vi "Main.vi"() -> ()   [LabVIEW 2013]
doc: "Diese Vorlage dient zur Erzeugung eines Entwurfsmusters für einen einfachen Zustandsautomaten. Jeder Zustand führt einen bestimmten Blockdiagrammabschnitt aus und ermittelt dann den nächsten Zustand."
uses:
  controls/State.ctl
  controls/Data.ctl
  res/classes/Datastructure/Report/Report.lvclass
  res/classes/Devices/emTestCWS500N/EMTestCWS500N.lvclass
  res/classes/Devices/CEG4500/CEG4500.lvclass
  res/classes/Devices/Tektronix RSA5106A/Tektronix RSA5106A.lvclass
  res/classes/Devices/DeviceInterface/Devices.ctl
  res/classes/Tests/TestInterface/Tests.ctl
  res/vis/Tabs.ctl
  res/vis/ESD Pistol.lvclass
  <vilib>/event_ctls.llb/eventvkey.ctl
  res/classes/Datastructure/Norm/Norm.lvclass
  res/classes/Datastructure/Test/Test.lvclass
  <vilib>/Utility/error.llb/DialogType.ctl
  res/classes/Datastructure/Setup/Setup.lvclass
  res/vis/DeviceAddEdit.vi
  res/vis/Versuchsaufbau bearbeiten.vi
  res/vis/Test bearbeiten.vi
  res/lib/DataCreation.lvlib
  res/lib/Utilities.lvlib
  res/lib/EMV-Test.lvlib
  res/lib/TreeRepresentation.lvlib
  res/lib/XML.lvlib
  res/lib/TempHygro.lvlib
panel:
  out "running":bool=TRUE
  in  "error in (no error)":errorcluster
  out "COM-Port Refs":refnum<vi>[](array[refnum])
  out "Normen":string[](array[string])
  out "APPDATA":string
  out "return code":i32 caption="Fehlercode"
  out "standard error":string caption="Standardfehler"
  out "standard output":string caption="Standardausgabe"
  in  "Tab Control":T1(tab)
  in  "Button:Beenden":bool
  in  "Button:Start:HF-Felder":bool
  in  "Button:Start:Spannungseinbruch":bool
  in  "Button:Start:Surge":bool
  in  "Button:Start:ESD":bool
  in  "Button:Start:Burst":bool
  in  "Button:Start:Störaussendung":bool
  in  "Button:save Report":bool caption="Blank Button"
  in  "Button:load Report":bool caption="Blank Button"
  in  "Button:create Pdf":bool caption="Blank Button"
  in  "Debug":bool
  in  "Tree":string(tree)
  in  "Bild-Qualität ( 0 = schlechteste, 1 = beste)":dbl(slide)=0.4954128440366973 min=0.0 max=1.0 scale=0.0..1.0
  in  "Kalibrierung CDN":bool
  in  "Tektronix RSA5106A":refnum<visa-resource-name>="COM4"
  in  "CEG 4500":refnum<visa-resource-name>="COM13"
  in  "emTestCWS500N1":refnum<visa-resource-name>="COM5"
  in  "wait until completion? (T)":bool=TRUE
  in  "Path":path=path "C:/Windows/System32"
  # "COM-Ports"
  # "Pdf-Report"
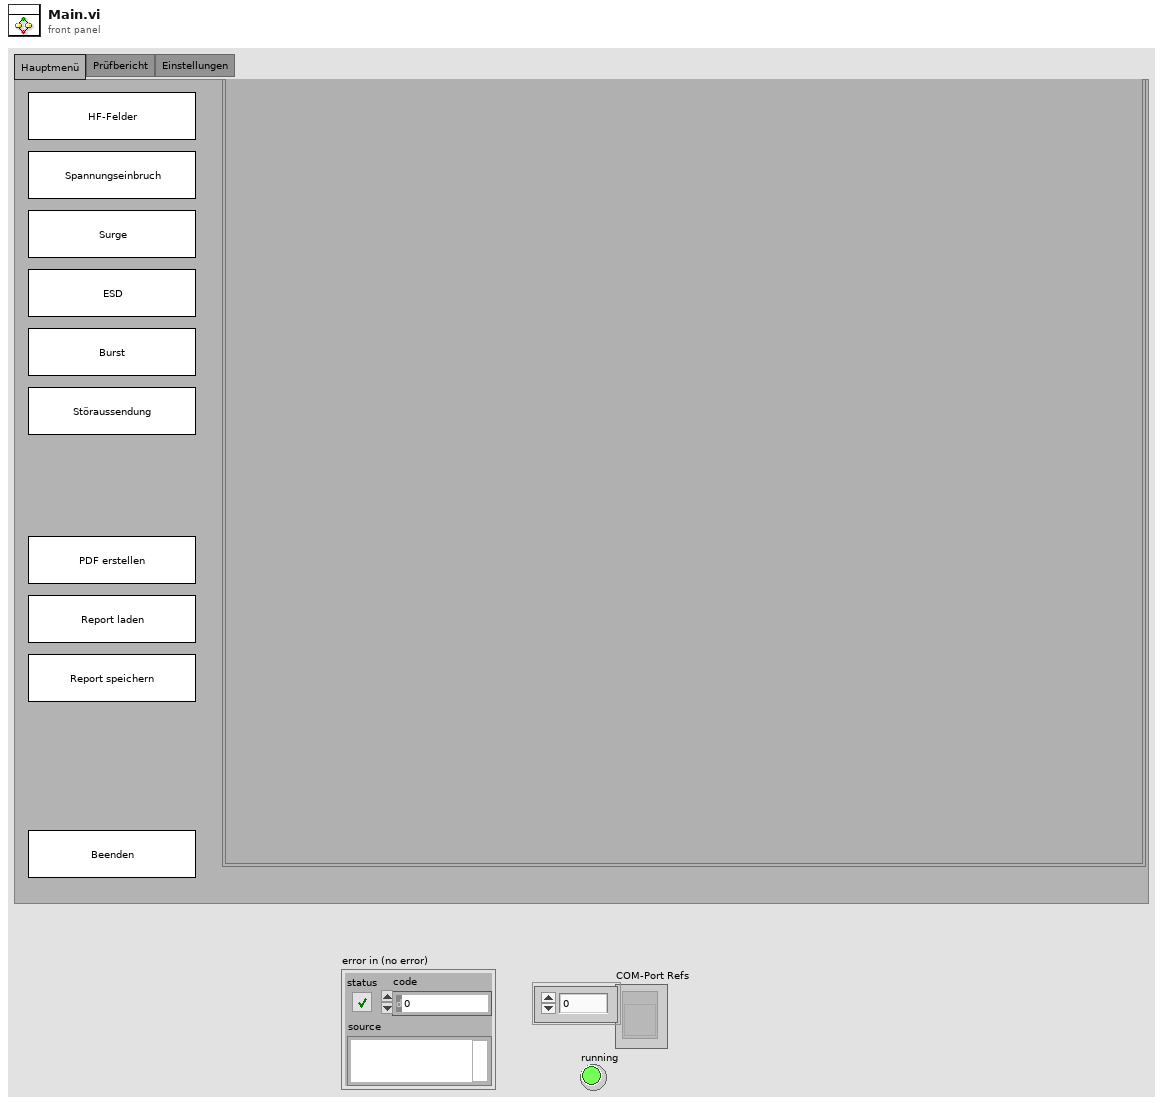
[diagram p1: front panel]
types:
  T1 = enum32{"Hauptmenü", "Prüfbericht", "Einstellungen"}
  T2 = typedef "Data.ctl" = cluster{"Report.lvclass":refnum<class "Report.lvclass">, "Norm":string, "last State":T3, "Norm ID":i32, "parameter":string[][], "EMTestCWS500N.lvclass":refnum<class "EMTestCWS500N.lvclass">, "CEG4500.lvclass":refnum<class "CEG4500.lvclass">, "Tektronix RSA5106A.lvclass":refnum<class "Tektronix RSA5106A.lvclass">, "erfolgreich":bool, "log":string, "Kommentar":string, "Device Enum":T4, "Test Enum":T5, "debug":bool, "tab":T6, "ESD Pistol.lvclass":refnum<class "ESD Pistol.lvclass">, "SubPnl Refnum":refnum<vi>, "TabCtl Refnum":refnum<vi>, "ButtonsEinblenden?":bool, "VKey":T7}
  T3 = typedef "State.ctl" = enum16{"create Pdf", "edit Report", "load Report", "save Report", "do Test", "CDN Kalibrierung", "enter Report Parameters", "new Test", "Protokoll", "read Tree", "update Tree", "Fehler", "Initialize", "Wait for Event", "Exit"}
  T4 = typedef "Devices.ctl" = enum16{"unbekannt", "ESD Pistol", "Tektronix RSA5106A", "emTestCWS500N", "CEG-4500"}
  T5 = typedef "Tests.ctl" = enum16{"unbekannt", "Störaussendung", "Burst", "ESD", "Surge", "Spannungseinbruch", "HF-Felder"}
  T6 = typedef "Tabs.ctl" = enum32{"Hauptmenü", "Prüfbericht", "Einstellungen"}
  T7 = typedef "eventvkey.ctl" = enum16{"ASCII", "Enter", "Return", "Shift", "Ctrl", "Alt", "Cmd", "Opt", "Caps", "NumLock", "Clear", "Break", "Up", "Down", "Left", "Right", "Insert", "Delete", "Home", "End", "PageUp", "PageDown", "Escape", "Help", "Pause", "ScrollLock", "F1", "F2", "F3", "F4", "F5", "F6", "F7", "F8", "F9", "F10", "F11", "F12", "F13", "F14", "F15", "F16", "F17", "F18", "F19", "F20", "F21", "F22", "F23", "F24", "Play", "VolumeUp", "VolumeDown", "Mute", "Two Byte Char"}
  T8 = enum8{"Enabled", "Disabled", "Disabled and Grayed Out"}
  T9 = typedef "DialogType.ctl" = u16
  T10 = enum16{"Left Button", "Center Button", "Right Button", "Window Close"}
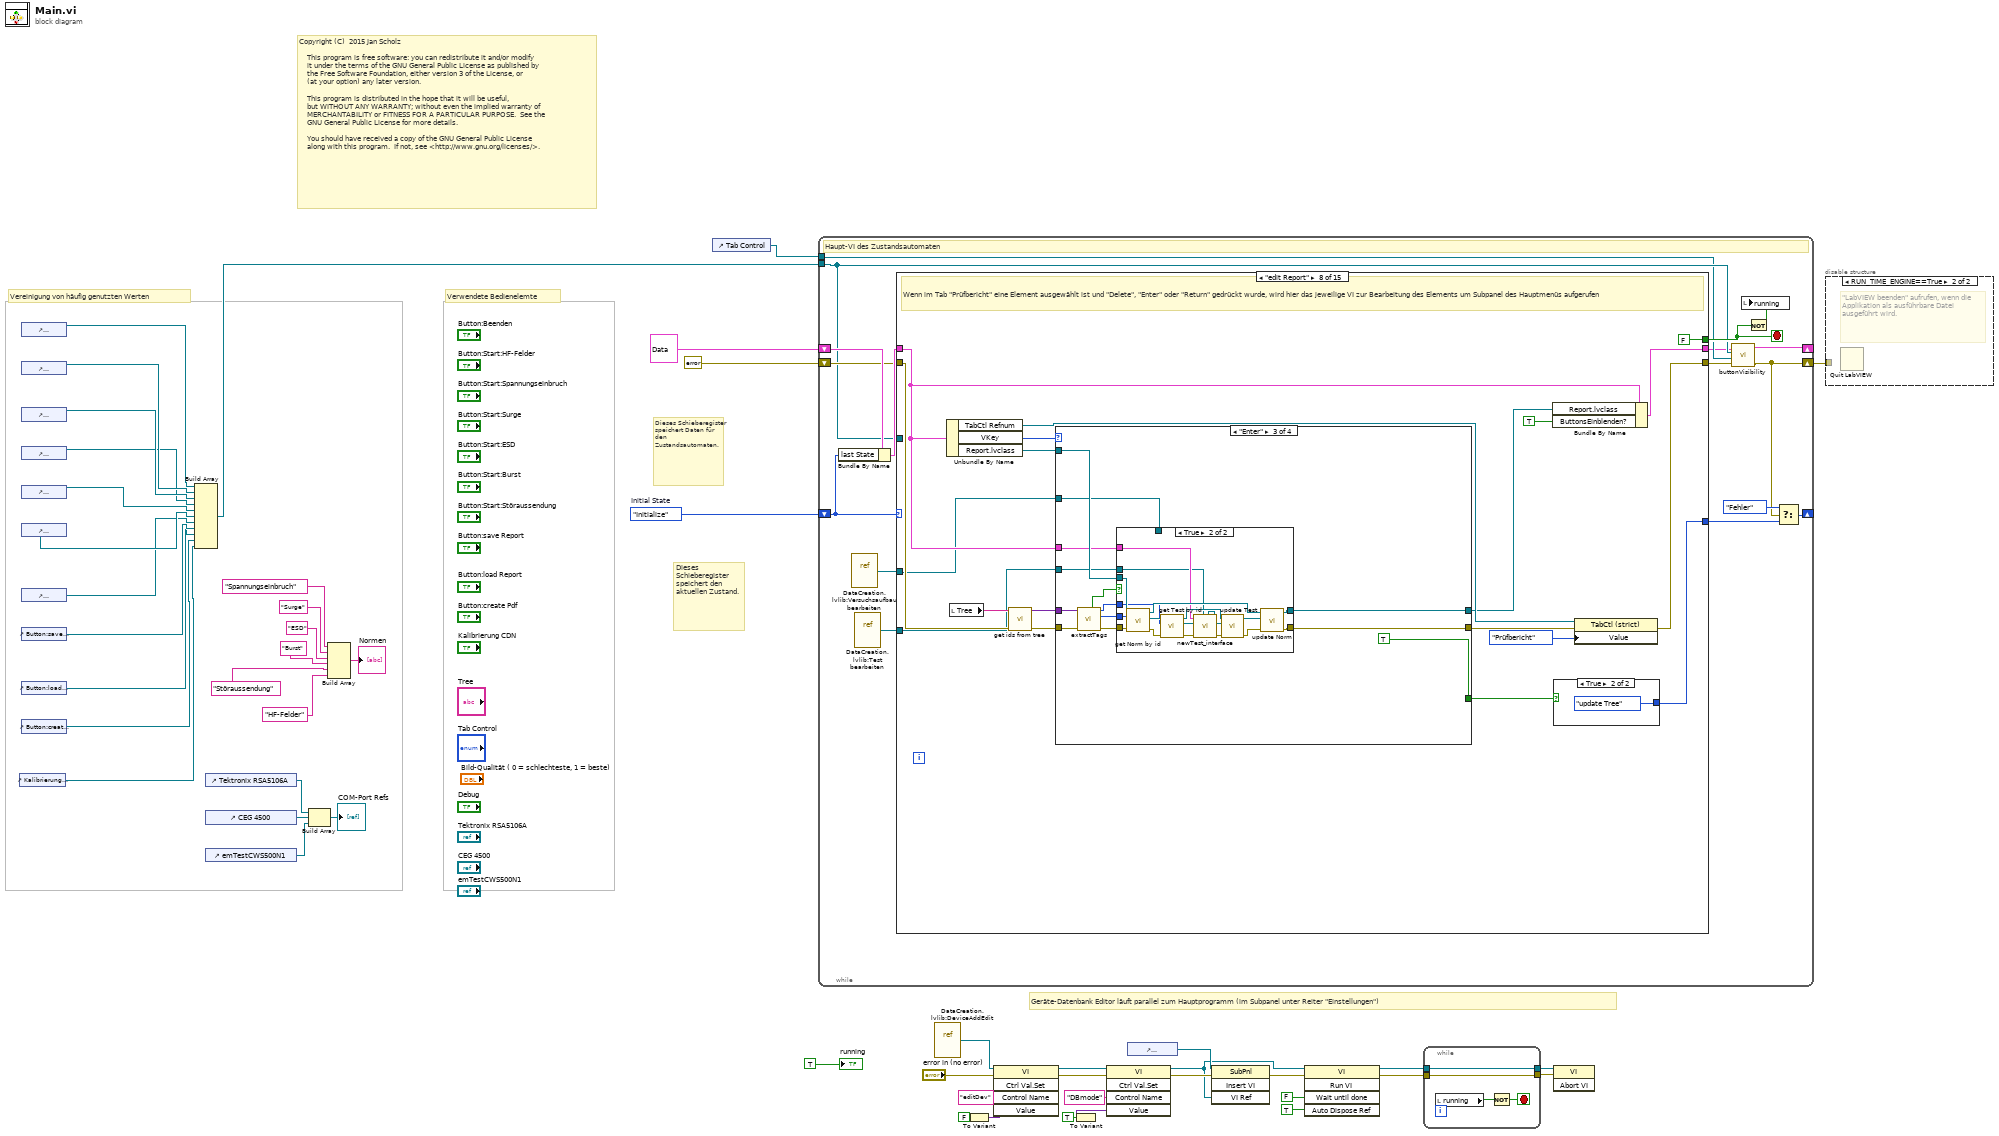
[diagram p0: block diagram]
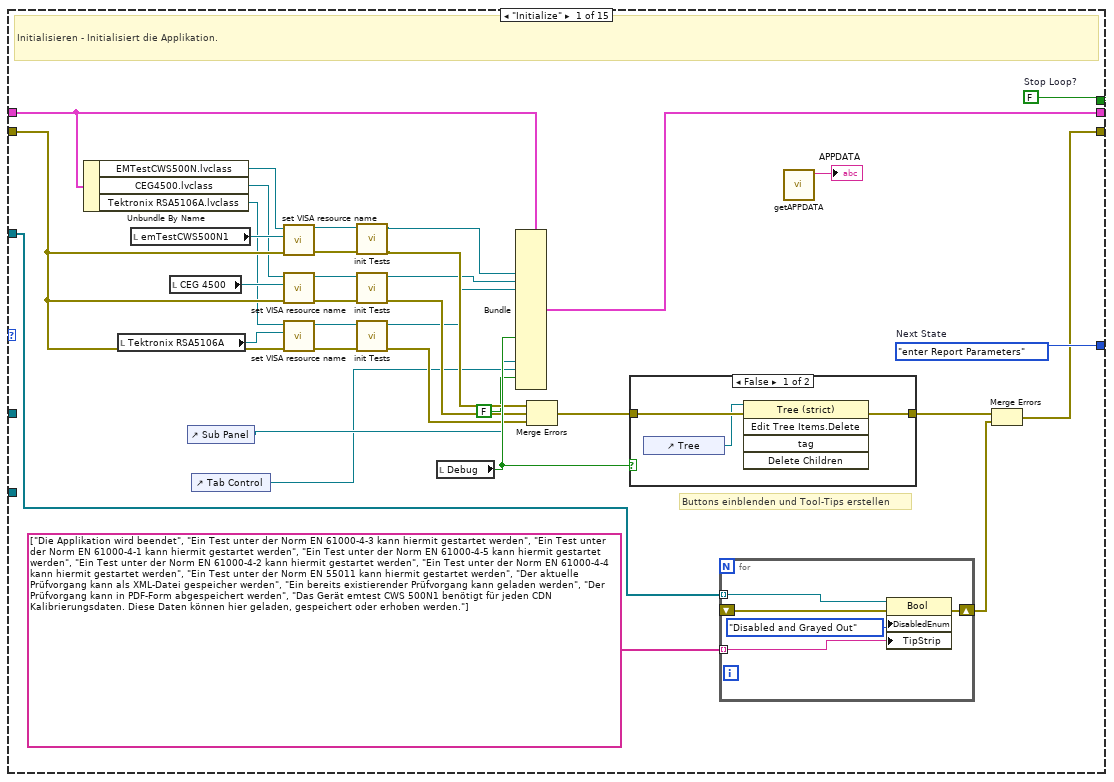
[diagram p3: hidden frame]
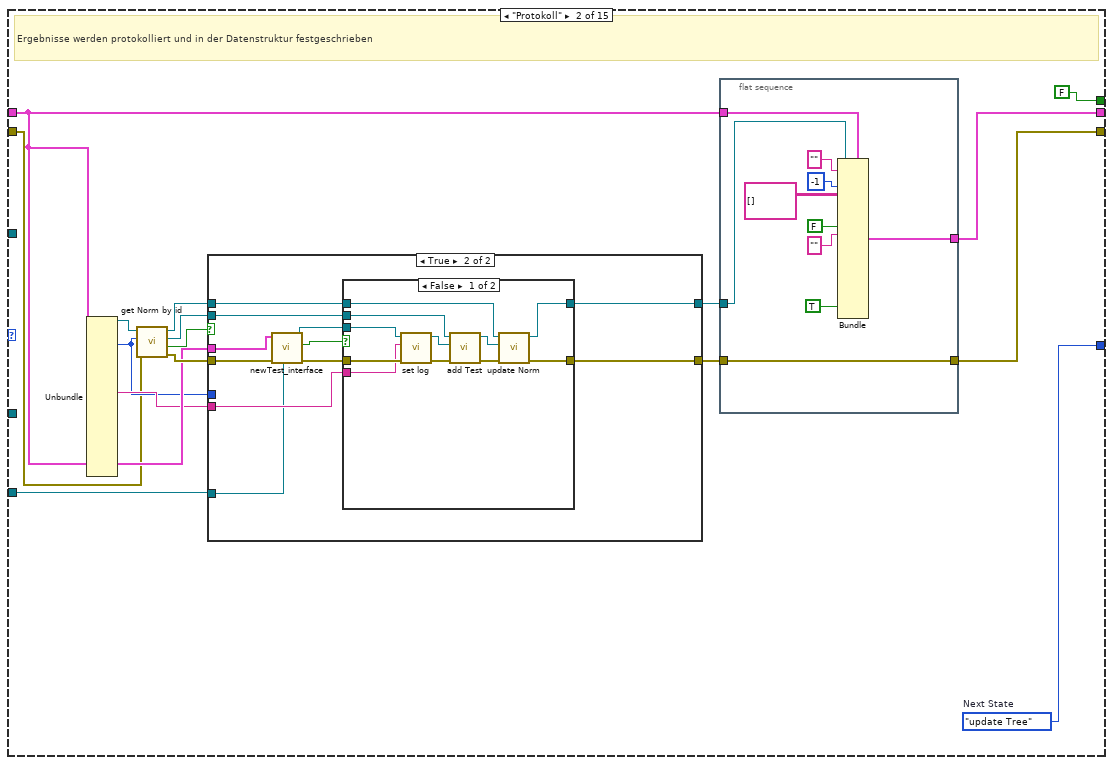
[diagram p5: hidden frame]
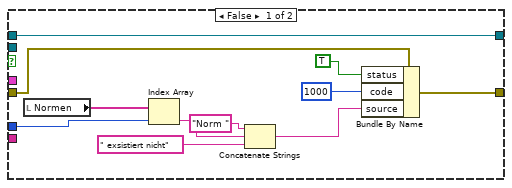
[diagram p6: hidden frame]
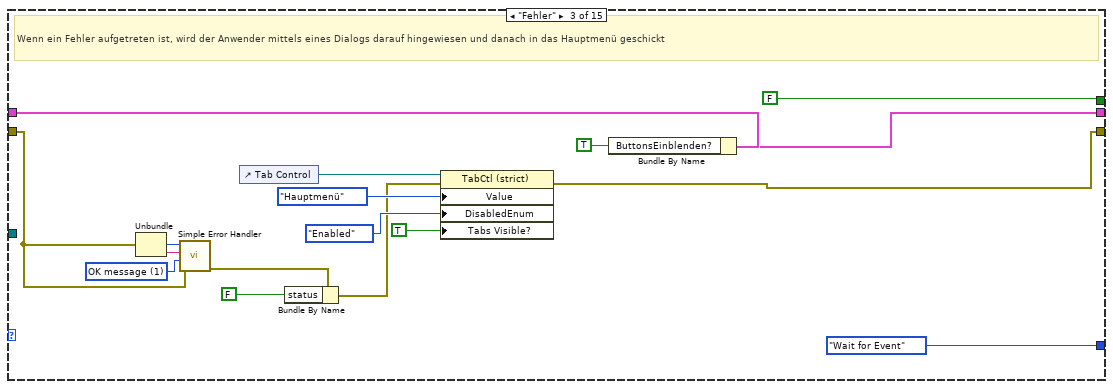
[diagram p8: hidden frame]
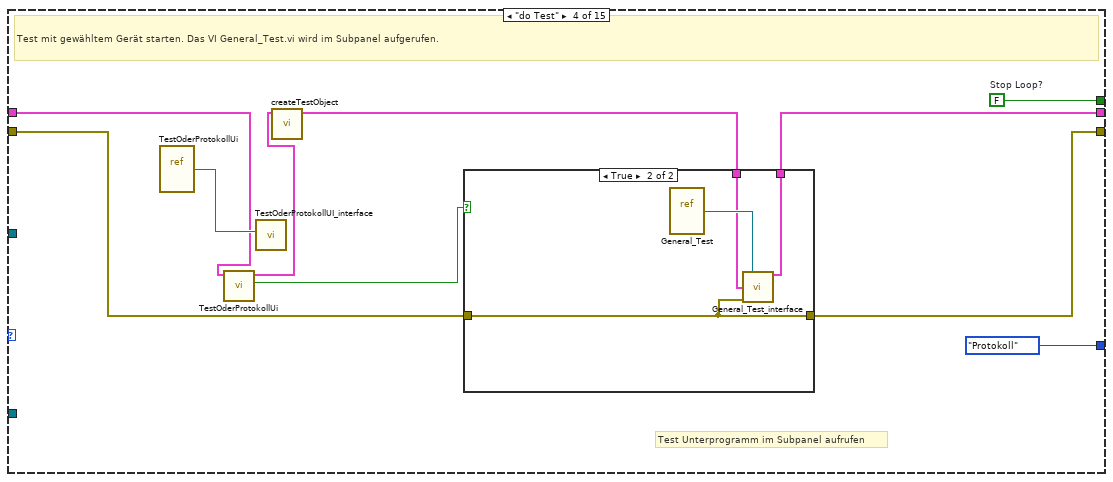
[diagram p9: hidden frame]
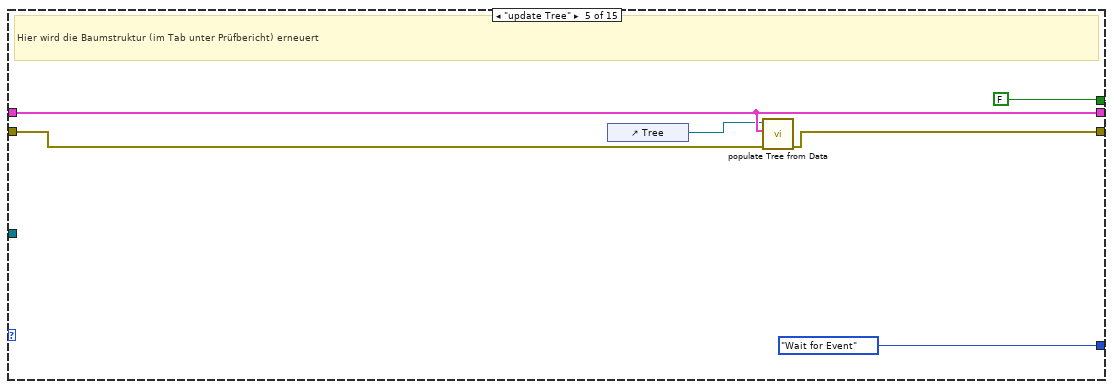
[diagram p11: hidden frame]
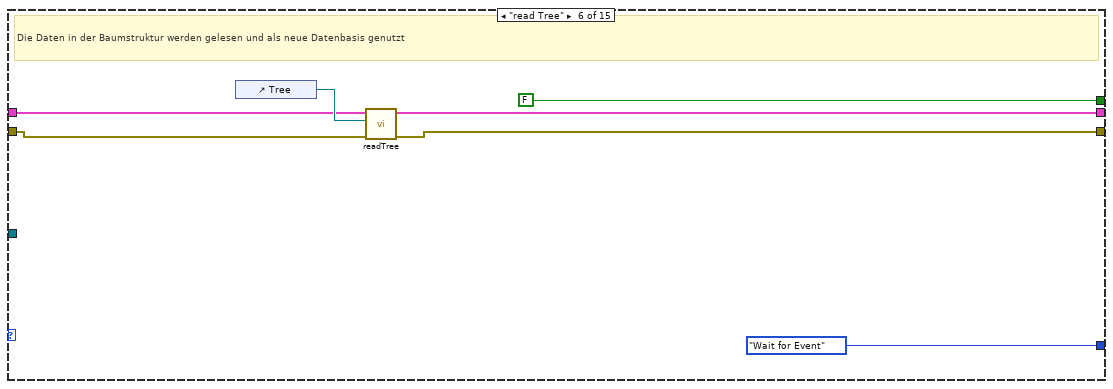
[diagram p12: hidden frame]
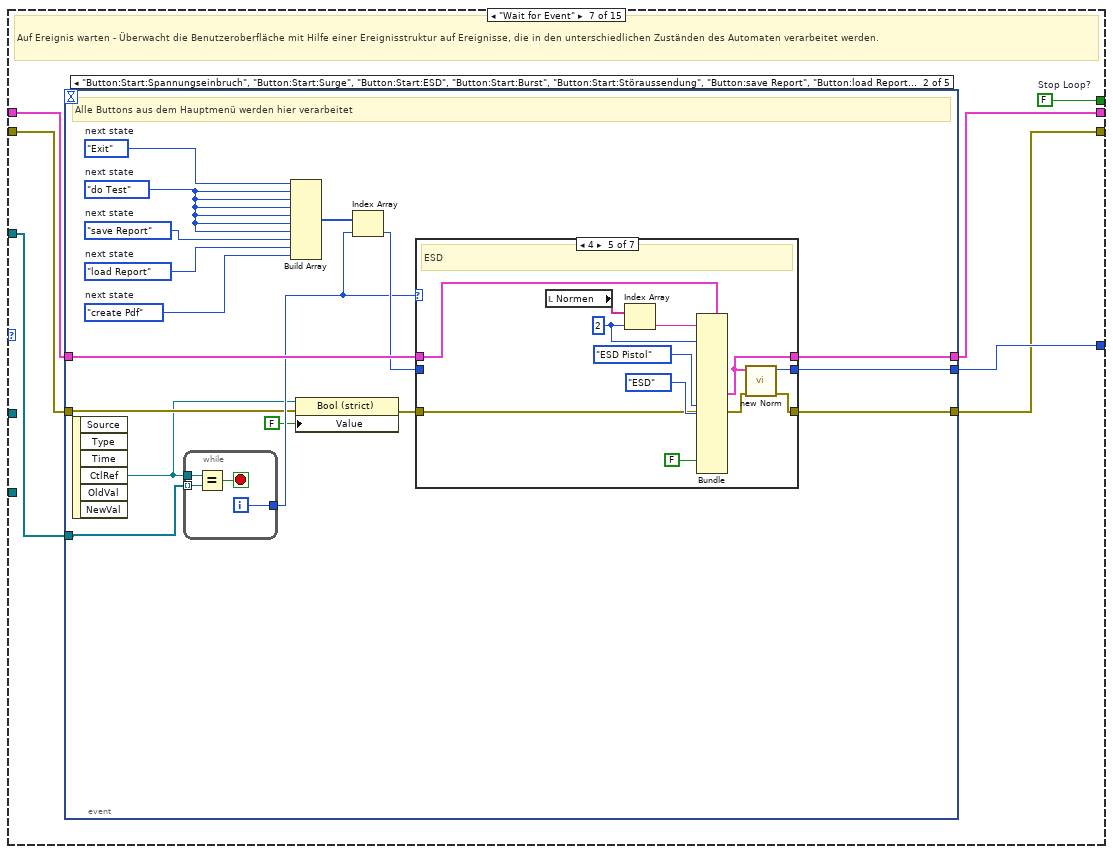
[diagram p13: hidden frame]
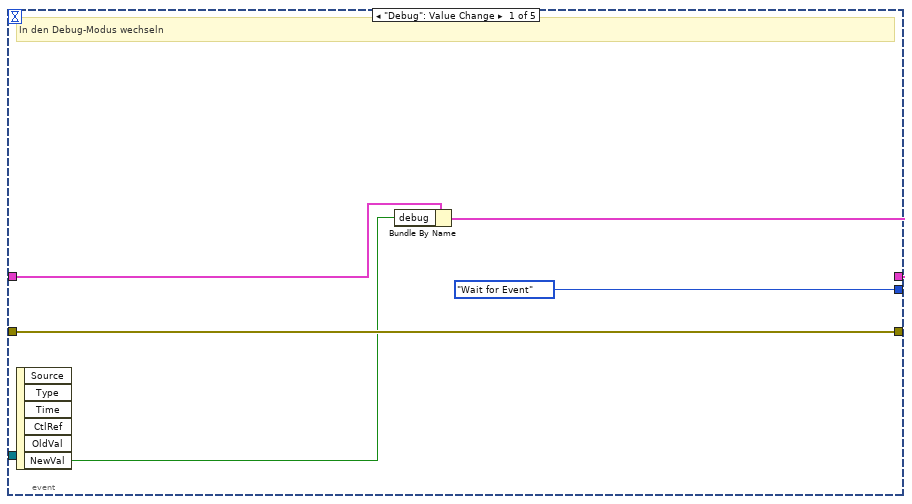
[diagram p14: hidden frame]
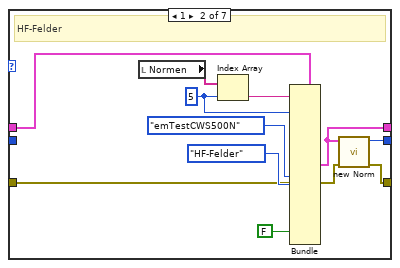
[diagram p16: hidden frame]
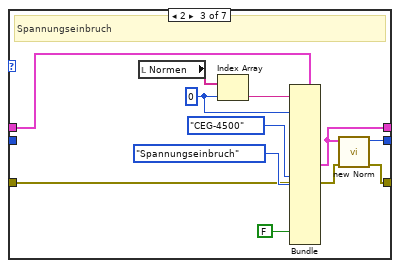
[diagram p17: hidden frame]
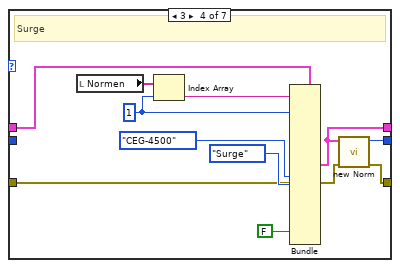
[diagram p18: hidden frame]
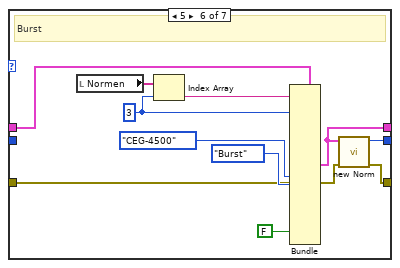
[diagram p19: hidden frame]
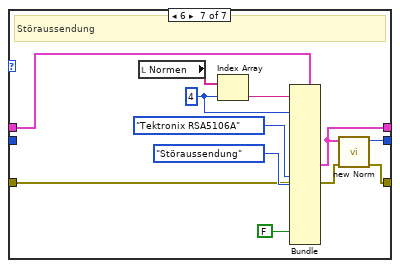
[diagram p20: hidden frame]
diagram:
  w46 = State."Initialize"  # Initial State
  # "Geräte-Datenbank Editor läuft parallel zum Hauptprogramm (im Subpanel unter Reiter \"Einstellungen\")"
  # "Copyright (C)  2015 Jan Scholz\n\n    This program is free software: you can redistribute it and/or modify\n    it under the terms of the GNU General Public License as published by\n    the Free Software Foundation, either version 3 of the License, or\n    (at your option) any later version.\n\n    This program is distributed in the hope that it will be useful,\n    but WITHOUT ANY WARRANTY; without even the implied warranty of\n    MERCHANTABILITY or FITNESS FOR A PARTICULAR PURPOSE.  See the\n    GNU General Public License for more details.\n\n    You should have received a copy of the GNU General Public License\n    along with this program.  If not, see <http://www.gnu.org/licenses/>."
  # "Vereinigung von häufig genutzten Werten"
  # "Verwendete Bedienelemte"
  # "Dieses Schieberegister speichert Daten für den Zustandsautomaten."
  # "Dieses Schieberegister speichert den aktuellen Zustand."
  n1 = control-ref of="Kalibrierung CDN"() -> (w24:refnum<vi>)
  n2 = control-ref of="Button:Beenden"() -> (w45:refnum<vi>)
  n3 = control-ref of="Button:Start:HF-Felder"() -> (w44:refnum<vi>)
  n4 = control-ref of="Button:Start:Spannungseinbruch"() -> (w43:refnum<vi>)
  n5 = control-ref of="Button:Start:Surge"() -> (w42:refnum<vi>)
  n6 = control-ref of="Button:Start:ESD"() -> (w41:refnum<vi>)
  n7 = control-ref of="Button:Start:Burst"() -> (w40:refnum<vi>)
  n8 = control-ref of="Button:Start:Störaussendung"() -> (w39:refnum<vi>)
  n9 = control-ref of="Button:save Report"() -> (w38:refnum<vi>)
  n10 = control-ref of="Button:load Report"() -> (w37:refnum<vi>)
  n11 = control-ref of="Button:create Pdf"() -> (w36:refnum<vi>)
  n12 = Build Array(w45, w44, w43, w42, w41, w40, w39, w38, w37, w36, w24) -> (w2:refnum<vi>[])
  n13 = control-ref of="Tektronix RSA5106A"() -> (w28:refnum<vi>)
  n14 = control-ref of="CEG 4500"() -> (w27:refnum<vi>)
  n15 = control-ref of="emTestCWS500N1"() -> (w26:refnum<vi>)
  n16 = Build Array(w28, w27, w26) -> (→"COM-Port Refs":refnum<vi>[])
  n17 = Build Array("Spannungseinbruch", "Surge", "ESD", "Burst", "Störaussendung", "HF-Felder") -> (→"Normen":string[])
  n18 = control-ref of="Tab Control"() -> (w1:refnum<vi>)
  n19 = while {
    shift-right: [w61] -> _
    shift-left: w46 -> [w65]
    shift-right: [w56] -> _
    shift-left: T2 {"Report.lvclass"=refnum, "Norm"="", "last State"=enum."create Pdf", "Norm ID"=0, "parameter"=[], "EMTestCWS500N.lvclass"=refnum, "CEG4500.lvclass"=refnum, "Tektronix RSA5106A.lvclass"=refnum, "erfolgreich"=FALSE, "log"="", "Kommentar"="", "Device Enum"=enum."unbekannt", "Test Enum"=enum."unbekannt", "debug"=FALSE, "tab"=enum."Hauptmenü", "ESD Pistol.lvclass"=refnum, "SubPnl Refnum"=refnum, "TabCtl Refnum"=refnum, "ButtonsEinblenden?"=FALSE, "VKey"=enum."ASCII"} ("Data") -> [w66]
    shift-right: [w57] -> w48
    shift-left: errorcluster {"status"=FALSE, "code"=0, "source"=""} ("error constant") -> [w55]
    tunnel: w2 -> [w54]
    tunnel: w1 -> [w53]
    stop <- w60 stop-if-true
    # "Haupt-VI des Zustandsautomaten"
    n20 = Bundle By Name(cluster=w66, "last State"=w65) -> (w64:T2)
    n21 = vi-ref "DataCreation.lvlib:Versuchsaufbau bearbeiten.vi"() -> (w52:refnum<vi>)
    n22 = vi-ref "DataCreation.lvlib:Test bearbeiten.vi"() -> (w51:refnum<vi>)
    n23 = case shown="\"edit Report\"" w65 {
      tunnel: [w99 w116 State."Wait for Event" ("Next State") State."Protokoll" ("Next State") State."Wait for Event" ("(Value Not Used)") State."Wait for Event" ("(Value Not Used)") w219 w398 State."Wait for Event" ("Next State") w599 State."Wait for Event" ("Next State") State."Wait for Event" ("(Value Not Used)") State."update Tree" ("Next State") w671 State."Wait for Event" ("f")] -> w63
      tunnel: [w100 FALSE FALSE w197 FALSE ("Stop Loop?") FALSE w223 FALSE ("Stop Loop?") FALSE ("Stop Loop?") w598 FALSE ("Stop Loop?") FALSE ("Stop Loop?") FALSE ("Stop Loop?") FALSE ("Stop Loop?") FALSE ("Stop Loop?")] -> w60
      tunnel: w64 -> [w90 w118 w173 w190 w207 w215 w222 w388 w590 w596 w604 w625 w637 w661 w710]
      tunnel: [w98 w124 w171 w196 w207 w210 w220 w385 w590 w596 w604 w623 w636 w672 w710] -> w50
      tunnel: w55 -> [w95 w114 w181 w193 w206 w214 w221 w394 w589 w597 w607 w629 w634 w660 w707]
      tunnel: [w83 w111 w174 w194 w208 w212 w218 w391 w588 w597 w606 w617 w635 w657 w709] -> w58
      tunnel: w54 -> [w67 _ _ _ _ _ w217 _ _ _ _ _ _ _ _]
      tunnel: w52 -> [_ _ _ _ _ _ _ w383 _ _ _ _ _ w655 _]
      tunnel: w51 -> [_ w113 _ _ _ _ _ w384 _ _ _ _ _ _ _]
      frame "Initialize" {
        w99 = State."enter Report Parameters"  # Next State
        w100 = FALSE  # Stop Loop?
        # "Buttons einblenden und Tool-Tips erstellen"
        # "Initialisieren - Initialisiert die Applikation."
        n24 = Unbundle By Name(w90) -> ("EMTestCWS500N.lvclass"=w89:refnum<class "EMTestCWS500N.lvclass">, "CEG4500.lvclass"=w88:refnum<class "CEG4500.lvclass">, "Tektronix RSA5106A.lvclass"=w87:refnum<class "Tektronix RSA5106A.lvclass">)
        n25 = local read "Tektronix RSA5106A"() -> (w92:refnum<visa-resource-name>)
        n26 = local read "emTestCWS500N1"() -> (w94:refnum<visa-resource-name>)
        n27 = local read "CEG 4500"() -> (w93:refnum<visa-resource-name>)
        n28 = control-ref of="Sub Panel"() -> (w70:refnum<vi>)
        n29 = control-ref of="Tab Control"() -> (w69:refnum<vi>)
        n30 = call-dynamic "set VISA resource name.vi"("error in (no error)"=w95, "VISA resource name"=w94, "DeviceInterface (Eingang)"=w89) -> ("error out"=w75:errorcluster, "DeviceInterface (Ausgang)"=w80:refnum<class "EMTestCWS500N.lvclass">)  [unwired: 7 in]
        n31 = call-dynamic "set VISA resource name.vi"("error in (no error)"=w95, "VISA resource name"=w93, "DeviceInterface (Eingang)"=w88) -> ("error out"=w76:errorcluster, "DeviceInterface (Ausgang)"=w77:refnum<class "CEG4500.lvclass">)  [unwired: 7 in]
        n32 = call-dynamic "set VISA resource name.vi"("error in (no error)"=w95, "VISA resource name"=w92, "DeviceInterface (Eingang)"=w87) -> ("error out"=w71:errorcluster, "DeviceInterface (Ausgang)"=w72:refnum<class "Tektronix RSA5106A.lvclass">)  [unwired: 7 in]
        n33 = call-dynamic "init Tests.vi"("error in (no error)"=w75, "EMTestCWS500N Eingang"=w80) -> ("error out"=w81:errorcluster, "EMTestCWS500N Ausgang"=w82:refnum<class "EMTestCWS500N.lvclass">)  [unwired: 8 in]
        n34 = call-dynamic "init Tests.vi"("error in (no error)"=w76, "CEG4500 Eingang"=w77) -> ("error out"=w78:errorcluster, "CEG4500 Ausgang"=w79:refnum<class "CEG4500.lvclass">)  [unwired: 8 in]
        n35 = call-dynamic "init Tests.vi"("error in (no error)"=w71, "Tektronix RSA5106A Eingang"=w72) -> ("error out"=w74:errorcluster, "Tektronix RSA5106A Ausgang"=w73:refnum<class "Tektronix RSA5106A.lvclass">)  [unwired: 8 in]
        n36 = local read "Debug"() -> (w91:bool)
        n37 = Bundle(cluster=w90, "EMTestCWS500N.lvclass"=w82, "CEG4500.lvclass"=w79, "Tektronix RSA5106A.lvclass"=w73, "debug"=w91, "SubPnl Refnum"=w70, "TabCtl Refnum"=w69, "ButtonsEinblenden?"=FALSE ("ButtonsAusblenden")) -> (w98:T2)  [unwired: 13 in]
        n38 = Merge Errors(w81, w78, w74) -> (w96:errorcluster)
        n39 = case shown="False" w91 {
          tunnel: [w103 w104] -> w85
          tunnel: w96 -> [w102 w104]
          frame False {
            n40 = control-ref of="Tree"() -> (w101:refnum<vi>)
            n41 = invoke on="Invoke Node" class="Tree (strict)" method="Edit Tree Items.Delete"(reference=w101, error in=w102) -> (error out=w103:errorcluster)  [unwired: 3 in, 4 out]
          }
          frame True {
          }
        }
        n42 = for {
          shift-right: [w107] -> w84
          shift-left: _ -> [w109]
          tunnel: w67 -> [w108] mode=indexing
          tunnel: string[] ["Die Applikation wird beendet", "Ein Test unter der Norm EN 61000-4-3 kann hiermit gestartet werden", "Ein Test unter der Norm EN 61000-4-1 kann hiermit gestartet werden", "Ein Test unter der Norm EN 61000-4-5 kann hiermit gestartet werden", "Ein Test unter der Norm EN 61000-4-2 kann hiermit gestartet werden", "Ein Test unter der Norm EN 61000-4-4 kann hiermit gestartet werden", "Ein Test unter der Norm EN 55011 kann hiermit gestartet werden", "Der aktuelle Prüfvorgang kann als XML-Datei gespeicher werden", "Ein bereits existierender Prüfvorgang kann geladen werden", "Der Prüfvorgang kann in PDF-Form abgespeichert werden", "Das Gerät emtest CWS 500N1 benötigt für jeden CDN Kalibrierungsdaten. Diese Daten können hier geladen, gespeichert oder erhoben werden."] -> [w105] mode=indexing
          n43 = property class="Bool"(reference=w108, error in=w109, "DisabledEnum"=T8."Disabled and Grayed Out" ("Deaktiviert"), "TipStrip"=w105) -> (error out=w107:errorcluster)  [unwired: 1 out]
        }
        n44 = call "getAPPDATA.vi"() -> ("APPDATA String/Binary data"=→"APPDATA":string)  [unwired: 11 in]
        n45 = Merge Errors(w85, w84) -> (w83:errorcluster)
      }
      frame "Protokoll" {
        w116 = State."update Tree"  # Next State
        # "Ergebnisse werden protokolliert und in der Datenstruktur festgeschrieben"
        n46 = Unbundle(w118) -> ("Report.lvclass"=w110:refnum<class "Report.lvclass">, "Norm ID"=w115:i32, "log"=w117:string)  [unwired: 17 out]
        n47 = call-dynamic "get Norm by id.vi"("error in (no error)"=w114, "id"=w115, "Report (Eingang)"=w110) -> ("error out"=w123:errorcluster, "id found"=w119:bool, "Norm.lvclass"=w122:refnum<class "Norm.lvclass">, "Report (Ausgang)"=w120:refnum<class "Report.lvclass">)  [unwired: 4 in, 1 out]
        n48 = case shown="True" w119 {
          tunnel: w123 -> [w144 w153]
          tunnel: w122 -> [_ w157]
          tunnel: [w145 w156] -> w112
          tunnel: [w146 w148] -> w121
          tunnel: w120 -> [w146 w147]
          tunnel: w115 -> [w140 _]
          tunnel: w118 -> [_ w154]
          tunnel: w117 -> [_ w155]
          tunnel: w113 -> [_ w149]
          frame False {
            n49 = local read "Normen"() -> (w141:string[])
            n50 = Index Array(array=w141, index=w140) -> (element=w138:string)
            n51 = Concatenate Strings("Norm " ("String"), w138, " exsistiert nicht" ("source")) -> (w136:string)
            n52 = Bundle By Name(cluster=w144, "status"=TRUE, "code"=1000, "source"=w136) -> (w145:errorcluster)
          }
          frame True {
            n53 = call "newTest_interface.vi"("Daten"=w154, "error in (no error)"=w153, "VI Refnum"=w149) -> ("Test.lvclass"=w152:refnum<class "Test.lvclass">, "abbrechen"=w151:bool, "error out"=w150:errorcluster)  [unwired: 5 in]
            n54 = case shown="False" w151 {
              tunnel: w157 -> [w168 _]
              tunnel: [w166 w170] -> w156
              tunnel: [w165 w169] -> w148
              tunnel: w147 -> [w164 w169]
              tunnel: w152 -> [w163 _]
              tunnel: w150 -> [w162 w170]
              tunnel: w155 -> [w160 _]
              frame False {
                n55 = call-dynamic "set log.vi"("error in (no error)"=w162, "log"=w160, "Test (Eingang)"=w163) -> ("error out"=w161:errorcluster, "Test (Ausgang)"=w159:refnum<class "Test.lvclass">)  [unwired: 7 in]
                n56 = call-dynamic "add Test.vi"("error in (no error)"=w161, "Test.lvclass"=w159, "Test Eingang"=w168) -> ("error out"=w167:errorcluster, "Test Ausgang"=w158:refnum<class "Norm.lvclass">)  [unwired: 7 in]
                n57 = call-dynamic "update Norm.vi"("error in (no error)"=w167, "Norm.lvclass"=w158, "Report in"=w164) -> ("error out"=w166:errorcluster, "Report out"=w165:refnum<class "Report.lvclass">)  [unwired: 7 in]
              }
              frame True {
              }
            }
          }
        }
        n58 = flat-sequence {
          tunnel: [w135] -> w124
          tunnel: w121 -> [w132]
          tunnel: w118 -> [w131]
          tunnel: w112 -> [w126]
          tunnel: [w126] -> w111
          frame #0 {
            n59 = Bundle(cluster=w131, "Report.lvclass"=w132, "Norm"="" ("test"), "Norm ID"=-1 ("test ID"), "parameter"=string[][] [], "erfolgreich"=FALSE, "log"="", "ButtonsEinblenden?"=TRUE ("ButtonsAusblenden")) -> (w135:T2)  [unwired: 13 in]
          }
        }
      }
      frame "Fehler" {
        w184 = T9 1 items=["no dialog", "OK message", "continue or stop message", "OK message + warnings", "continue/stop + warnings"] ("type of dialog (OK msg:1)")
        # "Wenn ein Fehler aufgetreten ist, wird der Anwender mittels eines Dialogs darauf hingewiesen und danach in das Hauptmenü geschickt"
        n60 = Unbundle(w181) -> ("code"=w183:i32, "source"=w182:string)  [unwired: 1 out]
        n61 = call <vilib>:"Simple Error Handler.vi"("error code (no error:0)"=w183, "error source (\" \")"=w182, "type of dialog (OK msg:1)"=w184, "error in (no error)"=w181) -> ("error out"=w186:errorcluster)  [unwired: 1 in, 4 out]
        n62 = control-ref of="Tab Control"() -> (w178:refnum<vi>)
        n63 = Bundle By Name(cluster=w186, "status"=FALSE) -> (w176:errorcluster)
        n64 = property class="TabCtl (strict)"(reference=w178, error in=w176, "Value"=T1."Hauptmenü" ("Value (Signaling)"), "DisabledEnum"=T8."Enabled" ("Deaktiviert"), "Tabs Visible?"=TRUE) -> (error out=w174:errorcluster)  [unwired: 1 out]
        n65 = Bundle By Name(cluster=w173, "ButtonsEinblenden?"=TRUE) -> (w171:T2)
      }
      frame "do Test" {
        w197 = FALSE  # Stop Loop?
        # "Test Unterprogramm im Subpanel aufrufen"
        # "Test mit gewähltem Gerät starten. Das VI General_Test.vi wird im Subpanel aufgerufen."
        n66 = vi-ref "TestOderProtokollUi.vi"() -> (w192:refnum<vi>)
        n67 = call "TestOderProtokollUi.vi"("Data in"=w190) -> ("TestMitGerät out"=w188:bool, "Data out"=w189:T2)  [unwired: 9 in]
        n68 = call "TestOderProtokollUI_interface.vi"("VI Refnum"=w192) -> ()  [unwired: 9 in, 2 out]
        n69 = call "createTestObject.vi"("Data in"=w189) -> ("Data out"=w191:T2)  [unwired: 10 in]
        n70 = case shown="True" w188 {
          tunnel: [w198 w202] -> w196
          tunnel: w191 -> [w198 w201]
          tunnel: w193 -> [w199 w200]
          tunnel: [w199 w200] -> w194
          frame False {
          }
          frame True {
            n71 = vi-ref "General_Test.vi"() -> (w203:refnum<vi>)
            n72 = call "General_Test_interface.vi"("VI Refnum"=w203, "Daten"=w201, "error in (no error)"=w200) -> ("Daten out"=w202:T2)  [unwired: 11 in, 1 out]
          }
        }
      }
      frame "update Tree" {
        # "Hier wird die Baumstruktur (im Tab unter Prüfbericht) erneuert"
        n73 = control-ref of="Tree"() -> (w205:refnum<vi>)
        n74 = call "populate Tree from Data.vi"("error in (no error)"=w206, "Data"=w207, "reference"=w205) -> ("error out"=w208:errorcluster)  [unwired: 6 in]
      }
      frame "read Tree" {
        # "Die Daten in der Baumstruktur werden gelesen und als neue Datenbasis genutzt"
        n75 = control-ref of="Tree"() -> (w216:refnum<vi>)
        n76 = call "readTree.vi"("Fehler (Eingang, kein Fehler)"=w214, "Tree ref"=w216, "Data out (Eingang)"=w215) -> ("error out"=w212:errorcluster, "Data out (Ausgang)"=w210:T2)  [unwired: 7 in]
      }
      frame "Wait for Event" {
        w223 = FALSE  # Stop Loop?
        # "Auf Ereignis warten - Überwacht die Benutzeroberfläche mit Hilfe einer Ereignisstruktur auf Ereignisse, die in den unterschiedlichen Zuständen des Automaten verarbeitet werden."
        n77 = event shown="[1] \"Button:Start:Spannungseinbruch\", \"Button:Start:Surge\", \"Button:Start:ESD\", \"Button:Start:Burst\", \"Button:Start:Störaussendung\", \"Button:save Report\", \"Button:load Report\", \"Button:create Pdf\", \"Button:Beenden\", \"Button:Start:HF-Felder\": Value Change" {
          selector: _ -> [_ _ _ _ _]
          dyn-events: _ -> [_ _ _ _ _]
          timeout: _ -> [_ _ _ _ _]
          tunnel: [State."Wait for Event" ("Next State") w238 State."CDN Kalibrierung" ("Next State") w331 State."Wait for Event" ("Next State")] -> w219
          tunnel: w222 -> [w227 w242 w321 w333 w347]
          tunnel: [w226 w240 w321 w326 w350] -> w220
          tunnel: w221 -> [w228 w232 w319 w329 w349]
          tunnel: [w228 w241 w319 w322 w348] -> w218
          tunnel: w217 -> [_ w229 _ _ _]
          event "Debug": Value Change {
            # "In den Debug-Modus wechseln"
            n78 = event-data() -> ("NewVal"=w224:bool)  [unwired: 1 in, 5 out]
            n79 = Bundle By Name(cluster=w227, "debug"=w224) -> (w226:T2)
          }
          event "Button:Start:Spannungseinbruch", "Button:Start:Surge", "Button:Start:ESD", "Button:Start:Burst", "Button:Start:Störaussendung", "Button:save Report", "Button:load Report", "Button:create Pdf", "Button:Beenden", "Button:Start:HF-Felder": Value Change {
            w235 = State."create Pdf"  # next state
            w236 = State."load Report"  # next state
            w237 = State."save Report"  # next state
            w244 = State."do Test"  # next state
            w245 = State."Exit"  # next state
            # "Alle Buttons aus dem Hauptmenü werden hier verarbeitet"
            n80 = event-data() -> ("CtlRef"=w231:refnum<vi>)  [unwired: 1 in, 5 out]
            n81 = while {
              tunnel: [w318] -> w234
              tunnel: w229 -> [w316] mode=indexing
              tunnel: w231 -> [w317]
              i -> [w318]
              stop <- w315 stop-if-true
              n82 = Equal?(x=w317, y=w316) -> (x = y?=w315:bool)
            }
            n83 = Build Array(w245, w244, w244, w244, w244, w244, w244, w237, w236, w235) -> (w243:T3[])
            n84 = property class="Bool (strict)"(reference=w231, error in=w232, "Value"=FALSE) -> (error out=w233:errorcluster)  [unwired: 1 out]
            n85 = Index Array(array=w243, index=w234) -> (element=w239:T3)
            n86 = case shown="4" w234 {
              tunnel: w233 -> [w247 w253 w265 w276 w286 w294 w308]
              tunnel: w242 -> [w248 w254 w264 w275 w287 w296 w309]
              tunnel: [w247 w252 w262 w273 w284 w297 w307] -> w241
              tunnel: [w248 w250 w261 w274 w283 w295 w305] -> w240
              tunnel: w239 -> [w246 _ _ _ _ _ _]
              tunnel: [w246 w251 w263 w272 w285 w298 w306] -> w238
              frame 0, Default {
                # "Beenden, Save, Load, Pdf, CDN Button"
              }
              frame 1 {
                w258 = 5 ("test ID")
                # "HF-Felder"
                n87 = local read "Normen"() -> (w259:string[])
                n88 = Index Array(array=w259, index=w258) -> (element=w257:string)
                n89 = Bundle(cluster=w254, "Norm"=w257, "Norm ID"=w258, "Device Enum"=Devices."emTestCWS500N", "Test Enum"=Tests."HF-Felder", "ButtonsEinblenden?"=FALSE ("ButtonsAusblenden")) -> (w250:T2)  [unwired: 15 in]
                n90 = call "new Norm.vi"("Fehler (Eingang, kein Fehler)"=w253, "Data"=w250) -> ("Fehler (Ausgang)"=w252:errorcluster, "Next State"=w251:T3)  [unwired: 8 in]
              }
              frame 2 {
                w269 = 0 ("test ID")
                # "Spannungseinbruch"
                n91 = local read "Normen"() -> (w270:string[])
                n92 = Index Array(array=w270, index=w269) -> (element=w268:string)
                n93 = Bundle(cluster=w264, "Norm"=w268, "Norm ID"=w269, "Device Enum"=Devices."CEG-4500", "Test Enum"=Tests."Spannungseinbruch", "ButtonsEinblenden?"=FALSE ("ButtonsAusblenden")) -> (w261:T2)  [unwired: 15 in]
                n94 = call "new Norm.vi"("Fehler (Eingang, kein Fehler)"=w265, "Data"=w261) -> ("Fehler (Ausgang)"=w262:errorcluster, "Next State"=w263:T3)  [unwired: 8 in]
              }
              frame 3 {
                w280 = 1 ("test ID")
                # "Surge"
                n95 = local read "Normen"() -> (w281:string[])
                n96 = Index Array(array=w281, index=w280) -> (element=w279:string)
                n97 = Bundle(cluster=w275, "Norm"=w279, "Norm ID"=w280, "Device Enum"=Devices."CEG-4500", "Test Enum"=Tests."Surge", "ButtonsEinblenden?"=FALSE ("ButtonsAusblenden")) -> (w274:T2)  [unwired: 15 in]
                n98 = call "new Norm.vi"("Fehler (Eingang, kein Fehler)"=w276, "Data"=w274) -> ("Fehler (Ausgang)"=w273:errorcluster, "Next State"=w272:T3)  [unwired: 8 in]
              }
              frame 4 {
                w292 = 2 ("test ID")
                # "ESD"
                n99 = local read "Normen"() -> (w290:string[])
                n100 = Index Array(array=w290, index=w292) -> (element=w291:string)
                n101 = Bundle(cluster=w287, "Norm"=w291, "Norm ID"=w292, "Device Enum"=Devices."ESD Pistol", "Test Enum"=Tests."ESD", "ButtonsEinblenden?"=FALSE ("ButtonsAusblenden")) -> (w283:T2)  [unwired: 15 in]
                n102 = call "new Norm.vi"("Fehler (Eingang, kein Fehler)"=w286, "Data"=w283) -> ("Fehler (Ausgang)"=w284:errorcluster, "Next State"=w285:T3)  [unwired: 8 in]
              }
              frame 5 {
                w302 = 3 ("test ID")
                # "Burst"
                n103 = local read "Normen"() -> (w303:string[])
                n104 = Index Array(array=w303, index=w302) -> (element=w301:string)
                n105 = Bundle(cluster=w296, "Norm"=w301, "Norm ID"=w302, "Device Enum"=Devices."CEG-4500", "Test Enum"=Tests."Burst", "ButtonsEinblenden?"=FALSE ("ButtonsAusblenden")) -> (w295:T2)  [unwired: 15 in]
                n106 = call "new Norm.vi"("Fehler (Eingang, kein Fehler)"=w294, "Data"=w295) -> ("Fehler (Ausgang)"=w297:errorcluster, "Next State"=w298:T3)  [unwired: 8 in]
              }
              frame 6 {
                w313 = 4 ("test ID")
                # "Störaussendung"
                n107 = local read "Normen"() -> (w314:string[])
                n108 = Index Array(array=w314, index=w313) -> (element=w312:string)
                n109 = Bundle(cluster=w309, "Norm"=w312, "Norm ID"=w313, "Device Enum"=Devices."Tektronix RSA5106A", "Test Enum"=Tests."Störaussendung", "ButtonsEinblenden?"=FALSE ("ButtonsAusblenden")) -> (w305:T2)  [unwired: 15 in]
                n110 = call "new Norm.vi"("Fehler (Eingang, kein Fehler)"=w308, "Data"=w305) -> ("Fehler (Ausgang)"=w307:errorcluster, "Next State"=w306:T3)  [unwired: 8 in]
              }
            }
          }
          event "Kalibrierung CDN": Value Change {
            n111 = event-data() -> ()  [unwired: 1 in, 6 out]
          }
          event "Tree": Key Down {
            # "Ist ein Element aus dem Tree ausgewählt und \"Return,Enter,Delete\" wird gedrückt kann der Datensatz gelöscht/geändert werden"
            n112 = event-data() -> ("VKey"=w332:T7)  [unwired: 1 in, 9 out]
            n113 = Bundle By Name(cluster=w333, "VKey"=w332) -> (w327:T2)
            n114 = control-ref of="Tab Control"() -> (w330:refnum<vi>)
            n115 = property class="TabCtl (strict)"(reference=w330, error in=w329) -> (reference out=w324:refnum<vi>, error out=w323:errorcluster, "Value"=w328:T1)
            n116 = case shown="\"Prüfbericht\"" w328 {
              tunnel: [State."Wait for Event" ("Next State") State."edit Report" ("Next State")] -> w331
              tunnel: [TRUE ("ButtonsEinblenden?") FALSE ("ButtonsEinblenden?")] -> w325
              tunnel: w324 -> [_ w340]
              tunnel: w323 -> [w334 w339]
              tunnel: [w334 w338] -> w322
              frame "Hauptmenü", Default {
              }
              frame "Prüfbericht" {
                n117 = property class="TabCtl (strict)"(reference=w340, error in=w339, "Value"=T1."Hauptmenü") -> (error out=w338:errorcluster)  [unwired: 1 out]
              }
            }
            n118 = Bundle By Name(cluster=w327, "ButtonsEinblenden?"=w325) -> (w326:T2)
          }
          event "emTestCWS500N1", "CEG 4500", "Tektronix RSA5106A": Value Change {
            # "Wenn die Com-Ports in den Einstellungen verändert werden, wird der neue COM-Port hier an das Gerät geknüpft"
            n119 = event-data() -> ("CtlRef"=w343:refnum<vi>, "NewVal"=w351:refnum<visa-resource-name>)  [unwired: 1 in, 4 out]
            n120 = local read "COM-Port Refs"() -> (w345:refnum<vi>[])
            n121 = Array Size(array=w345) -> (size(s)=w344:i32)
            n122 = while {
              tunnel: w343 -> [w381]
              tunnel: w345 -> [w382] mode=indexing
              tunnel: [w379] -> w352
              tunnel: w344 -> [w380]
              i -> [w379]
              stop <- w378 stop-if-true
              n123 = Equal?(x=w382, y=w381) -> (x = y?=w376:bool)
              n124 = Greater Or Equal?(x=w379, y=w380) -> (x >= y?=w377:bool)
              n125 = Or(x=w376, y=w377) -> (x .or. y?=w378:bool)
            }
            n126 = case shown="1" w352 {
              tunnel: w347 -> [w357 w360 w371 w375]
              tunnel: w351 -> [w353 w364 w372 _]
              tunnel: [w358 w361 w369 w375] -> w350
              tunnel: w349 -> [w355 w363 w368 _]
              tunnel: [w354 w362 w367 errorcluster {"status"=TRUE, "code"=6301, "source"="Die Änderung des COM-Ports konnte nicht festgeschrieben werden"} ("Fehlerkonstante")] -> w348
              frame 0 {
                n127 = Unbundle By Name(w357) -> ("Tektronix RSA5106A.lvclass"=w356:refnum<class "Tektronix RSA5106A.lvclass">)
                n128 = call-dynamic "set VISA resource name.vi"("error in (no error)"=w355, "VISA resource name"=w353, "DeviceInterface (Eingang)"=w356) -> ("error out"=w354:errorcluster, "DeviceInterface (Ausgang)"=w359:refnum<class "Tektronix RSA5106A.lvclass">)  [unwired: 7 in]
                n129 = Bundle By Name(cluster=w357, "Tektronix RSA5106A.lvclass"=w359) -> (w358:T2)
              }
              frame 1 {
                n130 = Unbundle By Name(w360) -> ("CEG4500.lvclass"=w365:refnum<class "CEG4500.lvclass">)
                n131 = call-dynamic "set VISA resource name.vi"("error in (no error)"=w363, "VISA resource name"=w364, "DeviceInterface (Eingang)"=w365) -> ("error out"=w362:errorcluster, "DeviceInterface (Ausgang)"=w366:refnum<class "CEG4500.lvclass">)  [unwired: 7 in]
                n132 = Bundle By Name(cluster=w360, "CEG4500.lvclass"=w366) -> (w361:T2)
              }
              frame 2 {
                n133 = Unbundle By Name(w371) -> ("EMTestCWS500N.lvclass"=w373:refnum<class "EMTestCWS500N.lvclass">)
                n134 = call-dynamic "set VISA resource name.vi"("error in (no error)"=w368, "VISA resource name"=w372, "DeviceInterface (Eingang)"=w373) -> ("error out"=w367:errorcluster, "DeviceInterface (Ausgang)"=w370:refnum<class "EMTestCWS500N.lvclass">)  [unwired: 7 in]
                n135 = Bundle By Name(cluster=w371, "EMTestCWS500N.lvclass"=w370) -> (w369:T2)
              }
              frame 3, Default {
              }
            }
          }
        }
      }
      frame "edit Report" {
        # "Wenn im Tab \"Prüfbericht\" eine Element ausgewählt ist und \"Delete\", \"Enter\" oder \"Return\" gedrückt wurde, wird hier das jeweilige VI zur Bearbeitung des Elements um Subpanel des Hauptmenüs aufgerufen"
        n136 = Unbundle By Name(w388) -> ("TabCtl Refnum"=w390:refnum<vi>, "VKey"=w396:T7, "Report.lvclass"=w395:refnum<class "Report.lvclass">)
        n137 = local read "Tree"() -> (w401:string)
        n138 = call "get ids from tree.vi"("error in"=w394, "Tree"=w401) -> ("error out"=w397:errorcluster, "tags"=w399:variant)  [unwired: 8 in]
        n139 = case shown="\"Enter\"" w396 {
          tunnel: w395 -> [w403 w420 w494 w542]
          tunnel: w397 -> [w404 w416 w488 w536]
          tunnel: [w404 w419 w492 w540] -> w392
          tunnel: [w403 w418 w493 w541] -> w387
          tunnel: w399 -> [_ w414 w489 w535]
          tunnel: [FALSE TRUE TRUE TRUE] -> w400
          tunnel: w388 -> [_ _ w490 w538]
          tunnel: w383 -> [_ _ w483 w531]
          tunnel: w384 -> [_ _ w482 w530]
          frame "ASCII", Default {
          }
          frame "Delete" {
            n140 = call "extractTags.vi"("error in (no error)"=w416, "tags"=w414) -> ("error out"=w415:errorcluster, "Norm"=w413:i32, "Test"=w412:i32, "level"=w411:i32, "isTest?"=w409:bool, "img"=w410:i32)  [unwired: 3 in, 1 out]
            n141 = Two Button Dialog(message="Soll der Eintrag wirklich gelöscht werden?" ("T button name (\"OK\")"), 1:"Abbrechen" ("F button name (\"Cancel\")"), 2:"Ja" ("T button name (\"OK\")")) -> (T button?=w405:bool)
            n142 = case shown="True" w405 {
              tunnel: w420 -> [w422 w431]
              tunnel: w415 -> [w421 w430]
              tunnel: [w421 w429] -> w419
              tunnel: [w422 w428] -> w418
              tunnel: w413 -> [_ w427]
              tunnel: w412 -> [_ w426]
              tunnel: w411 -> [_ w425]
              tunnel: w410 -> [_ w424]
              tunnel: w409 -> [_ w423]
              frame False {
              }
              frame True {
                n143 = case shown="2" w425 {
                  tunnel: w431 -> [w433 w438 w447 w460]
                  tunnel: w430 -> [w432 w437 w449 w461]
                  tunnel: [w432 w436 w441 w457] -> w429
                  tunnel: [w433 w435 w442 w458] -> w428
                  tunnel: w427 -> [_ w434 w440 w452]
                  tunnel: w426 -> [_ _ w439 _]
                  tunnel: w424 -> [_ _ _ w451]
                  tunnel: w423 -> [_ _ _ w450]
                  frame 0, Default {
                  }
                  frame 1 {
                    n144 = call-dynamic "delete Norm.vi"("error in (no error)"=w437, "id"=w434, "Report (Eingang)"=w438) -> ("error out"=w436:errorcluster, "Report (Ausgang)"=w435:refnum<class "Report.lvclass">)  [unwired: 7 in]
                  }
                  frame 2 {
                    n145 = call-dynamic "get Norm by id.vi"("error in (no error)"=w449, "id"=w440, "Report (Eingang)"=w447) -> ("error out"=w448:errorcluster, "Norm.lvclass"=w446:refnum<class "Norm.lvclass">, "Report (Ausgang)"=w444:refnum<class "Report.lvclass">)  [unwired: 4 in, 2 out]
                    n146 = call-dynamic "delete Test.vi"("error in (no error)"=w448, "id"=w439, "Test Eingang"=w446) -> ("error out"=w443:errorcluster, "Test Ausgang"=w445:refnum<class "Norm.lvclass">)  [unwired: 7 in]
                    n147 = call-dynamic "update Norm.vi"("error in (no error)"=w443, "Norm.lvclass"=w445, "Report in"=w444) -> ("error out"=w441:errorcluster, "Report out"=w442:refnum<class "Report.lvclass">)  [unwired: 7 in]
                  }
                  frame 3 {
                    n148 = call-dynamic "get Norm by id.vi"("error in (no error)"=w461, "id"=w452, "Report (Eingang)"=w460) -> ("error out"=w456:errorcluster, "Norm.lvclass"=w455:refnum<class "Norm.lvclass">, "Report (Ausgang)"=w459:refnum<class "Report.lvclass">)  [unwired: 4 in, 2 out]
                    n149 = case shown="True" w450 {
                      tunnel: w456 -> [w471 w480]
                      tunnel: w455 -> [w470 w481]
                      tunnel: [w465 w475] -> w453
                      tunnel: [w463 w476] -> w454
                      tunnel: w451 -> [w462 w472]
                      frame False {
                        n150 = call-dynamic "get Setup.vi"("error in (no error)"=w471, "Norm (Eingang)"=w470) -> ("error out"=w469:errorcluster, "Setup.lvclass"=w468:refnum<class "Setup.lvclass">, "Norm (Ausgang)"=w464:refnum<class "Norm.lvclass">)  [unwired: 7 in]
                        n151 = call-dynamic "del img.vi"("error in (no error)"=w469, "id"=w462, "Setup in"=w468) -> ("error out"=w466:errorcluster, "Setup out"=w467:refnum<class "Setup.lvclass">)  [unwired: 7 in]
                        n152 = call "update Setup.vi"("error in (no error)"=w466, "updated Setup"=w467, "Norm in"=w464) -> ("error out"=w465:errorcluster, "Norm out"=w463:refnum<class "Norm.lvclass">)  [unwired: 7 in]
                      }
                      frame True {
                        n153 = call-dynamic "get Test by id.vi"("error in (no error)"=w480, "Norm in"=w481) -> ("error out"=w479:errorcluster, "Test.lvclass"=w478:refnum<class "Test.lvclass">, "Norm out"=w474:refnum<class "Norm.lvclass">)  [unwired: 7 in]
                        n154 = call-dynamic "del img.vi"("error in (no error)"=w479, "id"=w472, "Test in"=w478) -> ("error out"=w477:errorcluster, "Test out"=w473:refnum<class "Test.lvclass">)  [unwired: 7 in]
                        n155 = call-dynamic "update Test.vi"("error in (no error)"=w477, "updated Test"=w473, "Norm in"=w474) -> ("error out"=w475:errorcluster, "Norm out"=w476:refnum<class "Norm.lvclass">)  [unwired: 7 in]
                      }
                    }
                    n156 = call-dynamic "update Norm.vi"("error in (no error)"=w453, "Norm.lvclass"=w454, "Report in"=w459) -> ("error out"=w457:errorcluster, "Report out"=w458:refnum<class "Report.lvclass">)  [unwired: 7 in]
                  }
                }
              }
            }
          }
          frame "Enter" {
            n157 = call "extractTags.vi"("error in (no error)"=w488, "tags"=w489) -> ("error out"=w487:errorcluster, "Norm"=w486:i32, "Test"=w485:i32, "isTest?"=w484:bool)  [unwired: 3 in, 3 out]
            n158 = case shown="True" w484 {
              tunnel: w494 -> [w511 w529]
              tunnel: w487 -> [w510 w528]
              tunnel: [w508 w522] -> w493
              tunnel: [w507 w520] -> w492
              tunnel: w490 -> [w500 w515]
              tunnel: w486 -> [w501 w519]
              tunnel: w485 -> [_ w518]
              tunnel: w483 -> [w495 _]
              tunnel: w482 -> [_ w514]
              frame False {
                n159 = call-dynamic "get Norm by id.vi"("error in (no error)"=w510, "id"=w501, "Report (Eingang)"=w511) -> ("error out"=w505:errorcluster, "Norm.lvclass"=w506:refnum<class "Norm.lvclass">, "Report (Ausgang)"=w509:refnum<class "Report.lvclass">)  [unwired: 4 in, 2 out]
                n160 = call-dynamic "get Setup.vi"("error in (no error)"=w505, "Norm (Eingang)"=w506) -> ("error out"=w498:errorcluster, "Setup.lvclass"=w499:refnum<class "Setup.lvclass">, "Norm (Ausgang)"=w502:refnum<class "Norm.lvclass">)  [unwired: 7 in]
                n161 = call "Setupbearbeiten_interface.vi"("VI Refnum"=w495, "error in (no error)"=w498, "Setup in"=w499, "Daten"=w500) -> ("error out"=w496:errorcluster, "Setup out"=w497:refnum<class "Setup.lvclass">)  [unwired: 5 in, 1 out]
                n162 = call "update Setup.vi"("error in (no error)"=w496, "updated Setup"=w497, "Norm in"=w502) -> ("error out"=w504:errorcluster, "Norm out"=w503:refnum<class "Norm.lvclass">)  [unwired: 7 in]
                n163 = call-dynamic "update Norm.vi"("error in (no error)"=w504, "Norm.lvclass"=w503, "Report in"=w509) -> ("error out"=w507:errorcluster, "Report out"=w508:refnum<class "Report.lvclass">)  [unwired: 7 in]
              }
              frame True {
                n164 = call-dynamic "get Norm by id.vi"("error in (no error)"=w528, "id"=w519, "Report (Eingang)"=w529) -> ("error out"=w526:errorcluster, "Norm.lvclass"=w527:refnum<class "Norm.lvclass">, "Report (Ausgang)"=w523:refnum<class "Report.lvclass">)  [unwired: 4 in, 2 out]
                n165 = call-dynamic "get Test by id.vi"("error in (no error)"=w526, "id"=w518, "Norm in"=w527) -> ("error out"=w517:errorcluster, "Test.lvclass"=w516:refnum<class "Test.lvclass">, "Norm out"=w525:refnum<class "Norm.lvclass">)  [unwired: 6 in]
                n166 = call "newTest_interface.vi"("Daten"=w515, "Test in"=w516, "error in (no error)"=w517, "VI Refnum"=w514) -> ("Test.lvclass"=w512:refnum<class "Test.lvclass">, "error out"=w513:errorcluster)  [unwired: 4 in, 1 out]
                n167 = call-dynamic "update Test.vi"("error in (no error)"=w513, "updated Test"=w512, "Norm in"=w525) -> ("error out"=w521:errorcluster, "Norm out"=w524:refnum<class "Norm.lvclass">)  [unwired: 7 in]
                n168 = call-dynamic "update Norm.vi"("error in (no error)"=w521, "Norm.lvclass"=w524, "Report in"=w523) -> ("error out"=w520:errorcluster, "Report out"=w522:refnum<class "Report.lvclass">)  [unwired: 7 in]
              }
            }
          }
          frame "Return" {
            n169 = call "extractTags.vi"("error in (no error)"=w536, "tags"=w535) -> ("error out"=w533:errorcluster, "Norm"=w537:i32, "Test"=w534:i32, "isTest?"=w532:bool)  [unwired: 3 in, 3 out]
            n170 = case shown="False" w532 {
              tunnel: w542 -> [w559 w577]
              tunnel: w533 -> [w558 w576]
              tunnel: [w556 w570] -> w541
              tunnel: [w555 w568] -> w540
              tunnel: w538 -> [w548 w563]
              tunnel: w537 -> [w550 w566]
              tunnel: w534 -> [_ w567]
              tunnel: w531 -> [w543 _]
              tunnel: w530 -> [_ w562]
              frame False {
                n171 = call-dynamic "get Norm by id.vi"("error in (no error)"=w558, "id"=w550, "Report (Eingang)"=w559) -> ("error out"=w554:errorcluster, "Norm.lvclass"=w549:refnum<class "Norm.lvclass">, "Report (Ausgang)"=w557:refnum<class "Report.lvclass">)  [unwired: 4 in, 2 out]
                n172 = call-dynamic "get Setup.vi"("error in (no error)"=w554, "Norm (Eingang)"=w549) -> ("error out"=w546:errorcluster, "Setup.lvclass"=w547:refnum<class "Setup.lvclass">, "Norm (Ausgang)"=w551:refnum<class "Norm.lvclass">)  [unwired: 7 in]
                n173 = call "Setupbearbeiten_interface.vi"("VI Refnum"=w543, "error in (no error)"=w546, "Setup in"=w547, "Daten"=w548) -> ("error out"=w545:errorcluster, "Setup out"=w544:refnum<class "Setup.lvclass">)  [unwired: 5 in, 1 out]
                n174 = call "update Setup.vi"("error in (no error)"=w545, "updated Setup"=w544, "Norm in"=w551) -> ("error out"=w553:errorcluster, "Norm out"=w552:refnum<class "Norm.lvclass">)  [unwired: 7 in]
                n175 = call-dynamic "update Norm.vi"("error in (no error)"=w553, "Norm.lvclass"=w552, "Report in"=w557) -> ("error out"=w555:errorcluster, "Report out"=w556:refnum<class "Report.lvclass">)  [unwired: 7 in]
              }
              frame True {
                n176 = call-dynamic "get Norm by id.vi"("error in (no error)"=w576, "id"=w566, "Report (Eingang)"=w577) -> ("error out"=w574:errorcluster, "Norm.lvclass"=w575:refnum<class "Norm.lvclass">, "Report (Ausgang)"=w571:refnum<class "Report.lvclass">)  [unwired: 4 in, 2 out]
                n177 = call-dynamic "get Test by id.vi"("error in (no error)"=w574, "id"=w567, "Norm in"=w575) -> ("error out"=w564:errorcluster, "Test.lvclass"=w565:refnum<class "Test.lvclass">, "Norm out"=w573:refnum<class "Norm.lvclass">)  [unwired: 6 in]
                n178 = call "newTest_interface.vi"("Daten"=w563, "Test in"=w565, "error in (no error)"=w564, "VI Refnum"=w562) -> ("Test.lvclass"=w561:refnum<class "Test.lvclass">, "error out"=w560:errorcluster)  [unwired: 4 in, 1 out]
                n179 = call-dynamic "update Test.vi"("error in (no error)"=w560, "updated Test"=w561, "Norm in"=w573) -> ("error out"=w569:errorcluster, "Norm out"=w572:refnum<class "Norm.lvclass">)  [unwired: 7 in]
                n180 = call-dynamic "update Norm.vi"("error in (no error)"=w569, "Norm.lvclass"=w572, "Report in"=w571) -> ("error out"=w568:errorcluster, "Report out"=w570:refnum<class "Report.lvclass">)  [unwired: 7 in]
              }
            }
          }
        }
        n181 = Bundle By Name(cluster=w388, "Report.lvclass"=w387, "ButtonsEinblenden?"=TRUE ("ButtonsAusblenden")) -> (w385:T2)
        n182 = case shown="True" w400 {
          tunnel: [State."Wait for Event" ("Next State") State."update Tree" ("Next State")] -> w398
          frame False {
          }
          frame True {
          }
        }
        n183 = property class="TabCtl (strict)"(reference=w390, error in=w392, "Value"=T1."Prüfbericht") -> (error out=w391:errorcluster)  [unwired: 1 out]
      }
      frame "create Pdf" {
        # "Ein Prüfbericht im Pdf-Format wird aus den Report-Daten generiert"
        n184 = local read "Bild-Qualität ( 0 = schlechteste, 1 = beste)"() -> (w583:dbl)
        n185 = control-ref of="APPDATA"() -> (w592:refnum<vi>)
        n186 = call "create Pdf.vi"("Bild-Qualität ( 0 = schlechteste, 1 = beste) 2"=w583, "Data"=w590, "Fehler (Eingang, kein Fehler)"=w589, "wait until completion? (T)"="wait until completion? (T)", "Path"="Path", "String (Eingang)"=w592) -> ("Fehler (Ausgang)"=w588:errorcluster, "return code"=→"return code":i32, "standard error"=w581:string, "standard output"=w582:string)  [unwired: 2 in]
        "standard output" <- w582
        "standard error" <- w581
        n187 = Concatenate Strings(w582, w581) -> (w580:string)
        n188 = String Length(string=w580) -> (length=w585:i32)
        n189 = Greater Than 0?(x=w585) -> (x > 0?=w584:bool)
        n190 = case shown="True" w584 {
          tunnel: w580 -> [_ w595]
          frame False {
          }
          frame True {
            n191 = One Button Dialog(message=w595) -> ()  [unwired: 1 in, 1 out]
          }
        }
      }
      frame "Exit" {
        w598 = TRUE  # Stop Loop?
        w599 = State."Exit"  # (Value Not Used)
        # "Beenden - Schließt das Programm."
      }
      frame "save Report" {
        # "Der Report wird hier als XML-Datei abgespeichert"
        n192 = call "Dateidialog"("error in"=w607, "pattern (all files)"="*.xml", "pattern label"="Report speichern") -> ("selected path"=w609:path, "cancelled"=w601:bool, "error out"=w608:errorcluster)  [unwired: 9 in, 1 out]
        n193 = case shown="False" w601 {
          tunnel: w609 -> [w613 _]
          tunnel: w608 -> [w612 _]
          tunnel: [w611 errorcluster {"status"=FALSE, "code"=0, "source"=""} ("Fehler (Ausgang)")] -> w606
          tunnel: w604 -> [w610 _]
          frame False {
            n194 = call "Generate XML String from Report Class.vi"("error in (no error)"=w612, "Dateipfad (Dialog verwenden)"=w613, "Daten"=w610) -> ("Fehler (Ausgang)"=w611:errorcluster)  [unwired: 8 in]
          }
          frame True {
          }
        }
      }
      frame "enter Report Parameters" {
        # "Zum Start des Programms wird nach dem Namen des Prüfers, dem Namen und der Artikelnummer der Braugruppe gefragt"
        n195 = control-ref of="Tab Control"() -> (w624:refnum<vi>)
        n196 = property class="TabCtl (strict)"(reference=w624, error in=w629, "Tabs Visible?"=FALSE) -> (error out=w627:errorcluster)  [unwired: 1 out]
        n197 = property class="TabCtl (strict)"(reference=w624, error in=w629, "Val(Sgnl)"=T1."Hauptmenü" ("Value (Signaling)"), "DisabledEnum"=T8."Enabled" ("Deaktiviert")) -> (error out=w621:errorcluster)  [unwired: 1 out]
        n198 = control-ref of="Sub Panel"() -> (w619:refnum<vi>)
        n199 = vi-ref "Report init.vi"() -> (w618:refnum<vi>)
        n200 = Merge Errors(w627, w621) -> (w620:errorcluster)
        n201 = call "Report init interface.vi"("Fehler (Eingang, kein Fehler)"=w620, "VI Referenz"=w618, "SubPanel (Eingang)"=w619) -> ("Fehler (Ausgang)"=w617:errorcluster, "Report out"=w616:refnum<class "Report.lvclass">)  [unwired: 7 in]
        n202 = Bundle By Name(cluster=w625, "ButtonsEinblenden?"=TRUE, "Report.lvclass"=w616) -> (w623:T2)
      }
      frame "load Report" {
        # "Ein Prüfbericht wird hier von einer ausgewählten Datei des Anwenders geladen"
        n203 = call "File Dialog"("error in"=w634, "pattern (all files)"="*.xml") -> ("selected path"=w642:path, "exists"=w639:bool, "cancelled"=w638:bool, "error out"=w644:errorcluster)  [unwired: 10 in]
        n204 = Not(x=w639) -> (.not. x?=w640:bool)
        n205 = Or(x=w640, y=w638) -> (x .or. y?=w641:bool)
        n206 = case shown="False" w641 {
          tunnel: w637 -> [w651 w653]
          tunnel: [w649 errorcluster {"status"=FALSE, "code"=0, "source"=""} ("error out")] -> w635
          tunnel: [w648 w653] -> w636
          tunnel: w642 -> [w647 _]
          tunnel: w644 -> [w646 _]
          frame False {
            n207 = call "readFromXML.vi"("error in (no error)"=w646, "file path (use dialog)"=w647) -> ("error out"=w649:errorcluster, "Report (Ausgang)"=w650:refnum<class "Report.lvclass">)  [unwired: 8 in]
            n208 = Bundle(cluster=w651, "Report.lvclass"=w650, "ButtonsEinblenden?"=TRUE) -> (w648:T2)  [unwired: 18 in]
          }
          frame True {
          }
        }
      }
      frame "new Test" {
        # "neues Norm-Objekt"
        # "Sollte noch kein Test unter dieser Norm vollzogen worden sein wird hier ein Versuchsaufbau angelegt und der Test mit Klimadaten und Zeitstempel initialisiert"
        n209 = local read "Debug"() -> (w674:bool)
        n210 = case shown="False" w674 {
          tunnel: w660 -> [w691 w698]
          tunnel: [w695 w699] -> w679
          tunnel: [w694 w700] -> w678
          tunnel: [w690 w698] -> w677
          frame False {
            n211 = call "temp_hygro_main.vi"("error in"=w691) -> ("error out"=w690:errorcluster, "Temperatur"=w692:dbl, "luftfeuchtigkeit"=w693:dbl)  [unwired: 8 in]
            n212 = Number To Fractional String(number=w693, precision (6)=i16 1) -> (F-format string=w694:string)  [unwired: 2 in]
            n213 = Number To Fractional String(number=w692, precision (6)=i16 1) -> (F-format string=w695:string)  [unwired: 2 in]
          }
          frame True {
            n214 = call "temp_hygro(mock).vi"() -> ("temp"=w699:string, "humidity"=w700:string)  [unwired: 10 in]
          }
        }
        n215 = call "Setupbearbeiten_interface.vi"("VI Refnum"=w655, "error in (no error)"=w660, "Daten"=w661) -> ("error out"=w659:errorcluster, "Setup out"=w658:refnum<class "Setup.lvclass">, "Abbrechen out"=w656:bool)  [unwired: 6 in]
        n216 = Unbundle By Name(w661) -> ("Norm"=w685:string, "Norm ID"=w666:i32, "Report.lvclass"=w663:refnum<class "Report.lvclass">)
        n217 = call-dynamic "add Setup.vi"("error in (no error)"=w659, "Setup"=w658, "Test Eingang"=refnum<class "Norm.lvclass"> refnum ("Test.lvclass")) -> ("error out"=w676:errorcluster, "Test Ausgang"=w680:refnum<class "Norm.lvclass">)  [unwired: 7 in]
        n218 = Merge Errors(w677, w676) -> (w675:errorcluster)
        n219 = Less Than 0?(x=w666) -> (x < 0?=w667:bool)
        n220 = call-dynamic "set NormName.vi"("error in (no error)"=w675, "name"=w685, "Norm (Eingang)"=w680) -> ("error out"=w688:errorcluster, "Norm (Ausgang)"=w689:refnum<class "Norm.lvclass">)  [unwired: 7 in]
        n221 = Select(t=State."Wait for Event" ("f"), s=w667, f=State."do Test") -> (s? t:f=w669:T3)
        n222 = call-dynamic "set temp.vi"("error in (no error)"=w688, "temp"=w679, "Norm (Eingang)"=w689) -> ("error out"=w687:errorcluster, "Norm (Ausgang)"=w686:refnum<class "Norm.lvclass">)  [unwired: 7 in]
        n223 = Select(t=State."Wait for Event", s=w656, f=w669) -> (s? t:f=w671:T3)
        n224 = call-dynamic "set humidity.vi"("error in (no error)"=w687, "humidity"=w678, "Test (Eingang)"=w686) -> ("error out"=w683:errorcluster, "Test (Ausgang)"=w684:refnum<class "Norm.lvclass">)  [unwired: 7 in]
        n225 = call-dynamic "set id.vi"("error in (no error)"=w683, "id"=w666, "Test (Eingang)"=w684) -> ("error out"=w664:errorcluster, "Test (Ausgang)"=w682:refnum<class "Norm.lvclass">)  [unwired: 7 in]
        n226 = call-dynamic "add Norm.vi"("error in (no error)"=w664, "Norm.lvclass"=w682, "Report (Eingang)"=w663) -> ("error out"=w657:errorcluster, "Report (Ausgang)"=w654:refnum<class "Report.lvclass">)  [unwired: 7 in]
        n227 = Bundle By Name(cluster=w661, "Report.lvclass"=w654, "ButtonsEinblenden?"=w656) -> (w673:T2)
        n228 = Select(t=w661, s=w656, f=w673) -> (s? t:f=w672:T2)
      }
      frame "CDN Kalibrierung" {
        # "Für das Gerät emtest CWS 500N1 können Kalibrierungsdaten für CDN's hinterlegt werden. Diese können auf den Rechner heruntergeladen werden und so zu einem späteren Zeitpunkt wieder in das Gerät geladen werden."
        n229 = call <vilib>:"Three Button Dialog.vi"("Right Button Text (\"Cancel\")"="Abbrechen" ("Right Button Text (\"Cancel\")"), "Center Button Text (\"No\")"="Auslesen" ("F button name (\"Cancel\")"), "Left Button Text (\"Yes\")"="Einlesen" ("T button name (\"OK\")"), "message"="Möchten Sie einen Kalibrierung einlesen/auslesen ?") -> ("Which Button?"=w702:T10)  [unwired: 7 in]
        n230 = Unbundle(w710) -> ("EMTestCWS500N.lvclass"=w708:refnum<class "EMTestCWS500N.lvclass">)  [unwired: 19 out]
        n231 = case shown="\"Left Button\", Default" w702 {
          tunnel: w708 -> [w720 w728 _ _]
          tunnel: w707 -> [w718 w726 w729 w730]
          tunnel: [w717 w727 w729 w730] -> w709
          frame "Left Button", Default {
            n232 = call "File Dialog2"("error in"=w718) -> ("selected path"=w716:path, "exists"=w713:bool, "cancelled"=w714:bool, "error out"=w719:errorcluster)  [unwired: 11 in]
            n233 = Not(x=w713) -> (.not. x?=w715:bool)
            n234 = Or(x=w714, y=w715) -> (x .or. y?=w712:bool)
            n235 = case shown="False" w712 {
              tunnel: w720 -> [w724 _]
              tunnel: w719 -> [w723 w725]
              tunnel: [w722 w725] -> w717
              tunnel: w716 -> [w721 _]
              frame False {
                n236 = call "EinlesenVonKalibrierung.vi"("Error in"=w723, "file path (use dialog)"=w721, "EMTestCWS500N.lvclass"=w724) -> ("Error Out"=w722:errorcluster)  [unwired: 6 in, 2 out]
              }
              frame True {
              }
            }
          }
          frame "Center Button" {
            n237 = call "AuslesenVonKalibrierung.vi"("Error in"=w726, "EMTestCWS500N.lvclass"=w728) -> ("error out"=w727:errorcluster)  [unwired: 6 in, 2 out]
          }
          frame "Right Button" {
          }
          frame "Window Close" {
          }
        }
      }
    }
    n238 = call "buttonVisibility.vi"("error in"=w58, "reference"=w53, "Button Refs"=w54, "Data in"=w50) -> ("error out"=w57:errorcluster, "Data out"=w56:T2)  [unwired: 6 in]
    n239 = Not(x=w60) -> (.not. x?=w59:bool)
    n240 = local write "running"(w59) -> ()
    n241 = Select(t=State."Fehler", s=w57, f=w63) -> (s? t:f=w61:T3)
  }
  n242 = vi-ref "DataCreation.lvlib:DeviceAddEdit.vi"() -> (w18:refnum<vi>)
  n243 = To Variant(anything=FALSE ("Warten bis beendet")) -> (Variant=w22:variant)
  n244 = invoke class="VI" method="Ctrl Val.Set"(reference=w18, error in="error in (no error)", "Control Name"="editDev", "Value"=w22) -> (reference out=w12:refnum<vi>, error out=w11:errorcluster)  [unwired: 1 in, 3 out]
  n245 = To Variant(anything=TRUE ("Warten bis beendet")) -> (Variant=w10:variant)
  n246 = invoke class="VI" method="Ctrl Val.Set"(reference=w12, error in=w11, "Control Name"="DBmode", "Value"=w10) -> (reference out=w13:refnum<vi>, error out=w14:errorcluster)  [unwired: 1 in, 3 out]
  n247 = control-ref of="Geräte-Datenbank Subpanel"() -> (w19:refnum<vi>)
  n248 = invoke on="Invoke Node" class="SubPnl" method="Insert VI"(reference=w19, error in=w14, "VI Ref"=w13) -> (error out=w23:errorcluster)  [unwired: 1 in, 3 out]
  n249 = invoke on="Methodenknoten" class="VI" method="Run VI"(reference=w13, error in=w23, "Wait until done"=FALSE ("Warten bis beendet"), "Auto Dispose Ref"=TRUE ("Referenz automatisch schließen")) -> (reference out=w3:refnum<vi>, error out=w6:errorcluster)  [unwired: 1 in, 3 out]
  n250 = while {
    tunnel: [w733] -> w5
    tunnel: w6 -> [w733]
    tunnel: [w732] -> w4
    tunnel: w3 -> [w732]
    stop <- w731 stop-if-true
    n251 = local read "running"() -> (w734:bool)
    n252 = Not(x=w734) -> (.not. x?=w731:bool)
  }
  n253 = invoke on="Methodenknoten" class="VI" method="Abort VI"(reference=w4, error in=w5) -> ()  [unwired: 1 in, 3 out]
  n254 = disable-structure shown="RUN_TIME_ENGINE==True" {
    disable-tunnel: w48 -> [_ _]
    frame condition #0 (active) {
    }
    frame condition #1 {
      # "\"LabVIEW beenden\" aufrufen, wenn die Applikation als ausführbare Datei ausgeführt wird."
      n255 = Quit LabVIEW() -> ()  [unwired: 1 in]
    }
  }
  "running" <- TRUE ("running")
